vi "DecorationVisibility.vi"(8 "error in":errorcluster, 10 "Visible":bool, 11 "TabControl in":refnum<vi>) -> (0 "error out":errorcluster)   [LabVIEW 2017]
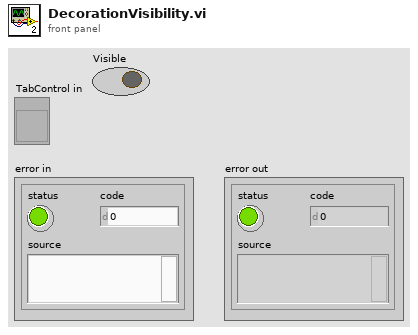
[diagram p1: front panel]
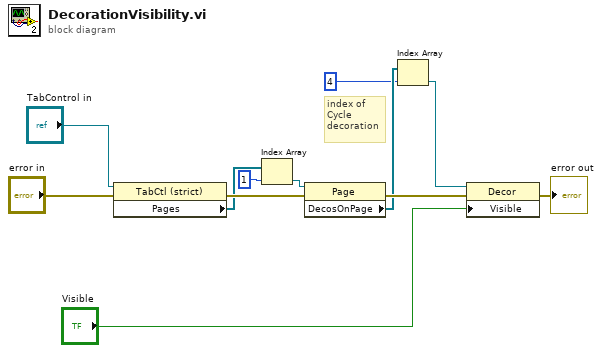
[diagram p0: block diagram]
diagram:
  # "index of \nCycle \ndecoration"
  n1 = property class="TabCtl (strict)"(reference="TabControl in", error in="error in") -> (error out=w10:errorcluster, "Pages"=w5:refnum<vi>[])  [unwired: 1 out]
  n2 = Index Array(array=w5, index=1) -> (element=w7:refnum<vi>)
  n3 = property class="Page"(reference=w7, error in=w10) -> (error out=w11:errorcluster, "DecosOnPage"=w8:refnum<vi>[])  [unwired: 1 out]
  n4 = Index Array(array=w8, index=4) -> (element=w2:refnum<vi>)
  n5 = property class="Decor"(reference=w2, error in=w11, "Visible"="Visible") -> (error out=→"error out":errorcluster)  [unwired: 1 out]
